vi "State Logic.vi"(9 "Filtering":bool, 10 "Processing":bool, 11 "Acquisition":bool) -> (3 "WhatToDo":string)   [LabVIEW 2020]
doc: "This VI is used for sending state or group of states to the queue depending on three main tasks, that can be turned ON or OFF in front panel. Inputs are boolean values, that indicate which task is ON and which is OFF."
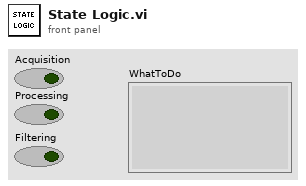
[diagram p1: front panel]
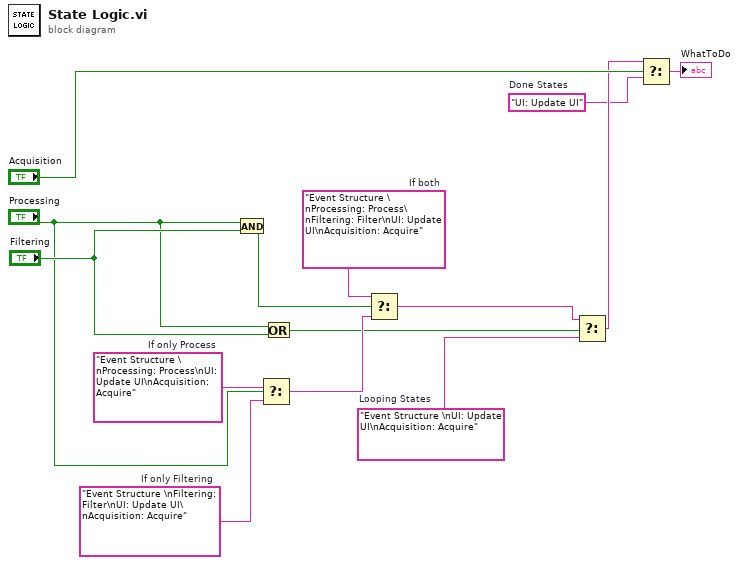
[diagram p0: block diagram]
diagram:
  w7 = "Event Structure \nUI: Update UI\nAcquisition: Acquire"  # Looping States
  w10 = "Event Structure \nFiltering: Filter\nUI: Update UI\nAcquisition: Acquire"  # If only Filtering
  w11 = "Event Structure \nProcessing: Process\nUI: Update UI\nAcquisition: Acquire"  # If only Process
  w13 = "Event Structure \nProcessing: Process\nFiltering: Filter\nUI: Update UI\nAcquisition: Acquire"  # If both
  w1 = "UI: Update UI"  # Done States
  n1 = And(x="Processing", y="Filtering") -> (x .and. y?=w14:bool)
  n2 = Select(t=w11, s="Processing", f=w10) -> (s? t:f=w12:string)
  n3 = Or(x="Processing", y="Filtering") -> (x .or. y?=w9:bool)
  n4 = Select(t=w13, s=w14, f=w12) -> (s? t:f=w8:string)
  n5 = Select(t=w8, s=w9, f=w7) -> (s? t:f=w2:string)
  n6 = Select(t=w2, s="Acquisition", f=w1) -> (s? t:f=→"WhatToDo":string)
